vi "RT_ShVariables.vi"   [LabVIEW 2019]
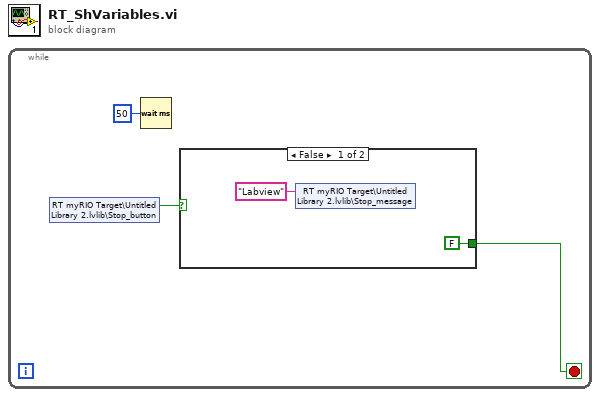
[diagram p0: block diagram]
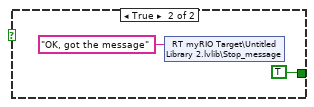
[diagram p2: hidden frame]
diagram:
  n1 = while {
    stop <- w2 stop-if-true
    n2 = shared-variable "RT myRIO Target\\Untitled Library 2.lvlib\\Stop_button"() -> (w3:bool)  [unwired: 1 in, 1 out]
    n3 = Wait (ms)(milliseconds to wait=u32 50) -> ()  [unwired: 1 out]
    n4 = case shown="False" w3 {
      tunnel: [FALSE TRUE] -> w2
      frame False {
        n5 = shared-variable "RT myRIO Target\\Untitled Library 2.lvlib\\Stop_message"("Labview" ("Variable4")) -> ()  [unwired: 1 in, 1 out]
      }
      frame True {
        n6 = shared-variable "RT myRIO Target\\Untitled Library 2.lvlib\\Stop_message"("OK, got the message" ("Stop_message")) -> ()  [unwired: 1 in, 1 out]
      }
    }
  }
